vi "Set BT INSTR TX.vi"(8 "error in (no error)":errorcluster, 10 "niDTS BT.lvlib:niDTS BT INSTR TX":refnum<class "niDTS BT INSTR TX.lvclass">, 11 "niDTS BT Tx Test in":refnum<class "niDTS BT Tx Test.lvclass">) -> (0 "error out":errorcluster, 3 "niDTS BT Tx Test out":refnum<class "niDTS BT Tx Test.lvclass">)   [LabVIEW 2015, in "niDTS BT.lvlib" / "niDTS BT Tx Test.lvclass"]
uses:
  niDTS BT Tx Test.lvclass
  Instrument/INSTR TX/niDTS BT INSTR TX.lvclass
  niDTS BT Tx Test.lvclass/niDTS BT Tx Test.ctl
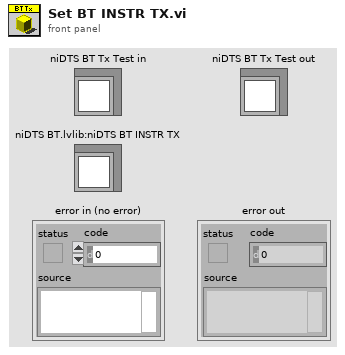
[diagram p1: front panel]
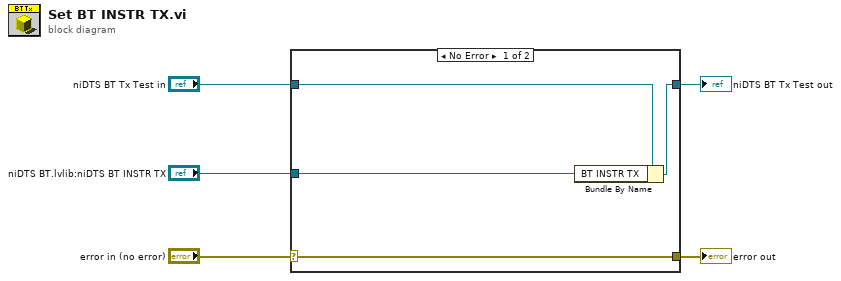
[diagram p0: block diagram]
diagram:
  n1 = case shown="No Error" "error in (no error)" {
    selector: "error in (no error)" -> [w9 w10]
    tunnel: [w9 w10] -> w4
    tunnel: [w7 w11] -> w2
    tunnel: "niDTS BT Tx Test in" -> [w8 w11]
    tunnel: "niDTS BT.lvlib:niDTS BT INSTR TX" -> [w6 _]
    frame No Error {
      n2 = Bundle By Name(cluster=w8, "BT INSTR TX"=w6) -> (w7:refnum<class "niDTS BT Tx Test.lvclass">)
    }
    frame Error {
    }
  }
  "error out" <- w4
  "niDTS BT Tx Test out" <- w2
